vi "PH_Beckhoff_PPMA-Rods.panel.vi"(0 "object ref":refnum<vi>, 5 "error in (no error)":errorcluster) -> (19 "error out":errorcluster)   [LabVIEW 2014, in "PH_Beckhoff_PPMA-Rods.lvlib"]
doc: "This a GUI.\n\nLicense Agreement for this software:\n\nCopyright (C)\nGesellschaft für Schwerionenforschung, GSI\nPlanckstr. 1\n64291 Darmstadt\nGermany\n\nContact: D.Beck@gsi.de \n\nThis program is free software; you can redistribute it and/or modify it under the terms of the GNU General Public License as published by the Free Software Foundation; either version 2 of the license, or (at your option) any later version.\n\nThis program is distributed in the hope that it will be useful, but WITHOUT ANYW ARRANTY; without even the implied warranty of MERCHANTABILITY or FITNESS FOR A PARTICULAR PURPOSE. See the GNU General License for more details (http://www.gnu.org).\n\nGesellschaft für Schwerionenforschung, GSI\nPlanckstr. 1, 64291 Darmstadt, Germany\nFor all questions and ideas contact: M.Richter@gsi.de, H.Brand@gsi.de or D.Beck@gsi.de.\nLast update: 18-DEC-2002"
uses:
  PH_Beckhoff_PPMA-Rods.lvlib
  PH_Beckhoff/PH_Beckhoff.Connectivity.ctl
  PH_Beckhoff/PH_Beckhoff.ADS Error.ctl
  PH_Beckhoff/PH_Beckhoff.Values.ctl
  PH_Beckhoff/PH_Beckhoff.Sonderklemmen Inputs.ctl
  PH_Beckhoff/PH_Beckhoff.Analog Inputs.ctl
  PH_Beckhoff/PH_Beckhoff.Scaling Type.ctl
  PH_Beckhoff/PH_Beckhoff.Analog Outputs.ctl
  PH_Beckhoff/PH_Beckhoff.Digital Inputs.ctl
  PH_Beckhoff/PH_Beckhoff.Digital Outputs.ctl
  PH_Basics/PH_StatusHandler/PH_StatusHandler.GUI element.ctl
  PH_Beckhoff/PH_Beckhoff.GUI Refs.ctl
  CS_Core/CSObj/CSObj.lvlib
  PH_Basics/PH_Common/PH_Common.lvlib
  PH_Beckhoff/PH_Beckhoff.lvlib
  CS_Core/CSSystem/CSSystemLib/CSSystemLib.lvlib
  PH_Basics/PH_Class/PH_Class.lvlib
  PH_Basics/PH_StatusHandler/PH_StatusHandler.lvlib
panel:
  in  "Tab Control":enum32{"Beckhoff Stuff", "Rods ..."}(tab)=enum."Rods ..."
  out "Current Values":T1
  out "ADS Error":T8
  out "IP":string
  out "Connection":T9
  out "configured?":bool
  out "Prdc Int [ms]":i32
  out "valve closed":u32(colorbox)
  out "door locked K2":u32(colorbox)
  out "door locked K1":u32(colorbox)
  out "earth ok":u32(colorbox)
  in  "Warnlamp green on":bool
  in  "Warnlamp orange on":bool
  out "PILC":T10 caption="Enabling State"
  out "FR":T10 caption="Enabling State"
  out "PU 6":T10 caption="Enabling State"
  out "PU 5":T10 caption="Enabling State"
  out "PU 4":T10 caption="Enabling State"
  out "PU 3":T10 caption="Enabling State"
  out "PU 2":T10 caption="Enabling State"
  out "PU 1":T10 caption="Enabling State"
  out "ROD 51":u32(colorbox)
  out "ROD 53":u32(colorbox)
  out "ROD 52":u32(colorbox)
  out "ROD 54":u32(colorbox)
  out "ROD 50":u32(colorbox)
  out "ROD 49":u32(colorbox)
  out "ROD 48":u32(colorbox)
  out "ROD 47":u32(colorbox)
  out "ROD 46":u32(colorbox)
  out "ROD 45":u32(colorbox)
  out "ROD 44":u32(colorbox)
  out "ROD 43":u32(colorbox)
  out "ROD 42":u32(colorbox)
  out "ROD 41":u32(colorbox)
  out "ROD 39":u32(colorbox)
  out "ROD 40":u32(colorbox)
  out "ROD 37":u32(colorbox)
  out "ROD 38":u32(colorbox)
  out "ROD 35":u32(colorbox)
  out "ROD 36":u32(colorbox)
  out "ROD 33":u32(colorbox)
  out "ROD 34":u32(colorbox)
  out "ROD 31":u32(colorbox)
  out "ROD 32":u32(colorbox)
  out "ROD 30":u32(colorbox)
  out "ROD 29":u32(colorbox)
  out "ROD 28":u32(colorbox)
  out "ROD 27":u32(colorbox)
  out "ROD 26":u32(colorbox)
  out "ROD 25":u32(colorbox)
  out "ROD 24":u32(colorbox)
  out "ROD 23":u32(colorbox)
  out "ROD 22":u32(colorbox)
  out "ROD 21":u32(colorbox)
  out "ROD 19":u32(colorbox)
  out "ROD 20":u32(colorbox)
  out "ROD 17":u32(colorbox)
  out "ROD 18":u32(colorbox)
  out "ROD 15":u32(colorbox)
  out "ROD 16":u32(colorbox)
  out "ROD 13":u32(colorbox)
  out "ROD 14":u32(colorbox)
  out "ROD 11":u32(colorbox)
  out "ROD 12":u32(colorbox)
  out "ROD 10":u32(colorbox)
  out "ROD 9":u32(colorbox)
  out "ROD 8":u32(colorbox)
  out "ROD 7":u32(colorbox)
  out "ROD 6":u32(colorbox)
  out "ROD 5":u32(colorbox)
  out "ROD 4":u32(colorbox)
  out "ROD 3":u32(colorbox)
  out "ROD 2":u32(colorbox)
  out "ROD 1":u32(colorbox)
  in  "rods_chain_b_up":bool
  in  "rods_chain_a_up":bool
  in  "Show Info":bool
  in  "Delete":bool
  in  "Exit":bool
  # "PCS"
  # "3.40"
  # "Pay attention! Commands are remote controlled! Handle with care!"
  # "B"
  # "A"
  # "B"
  # "A"
  # "A"
  # "B"
  # "B"
  # "A"
  # "A"
  # "B"
  # "A"
  # "B"
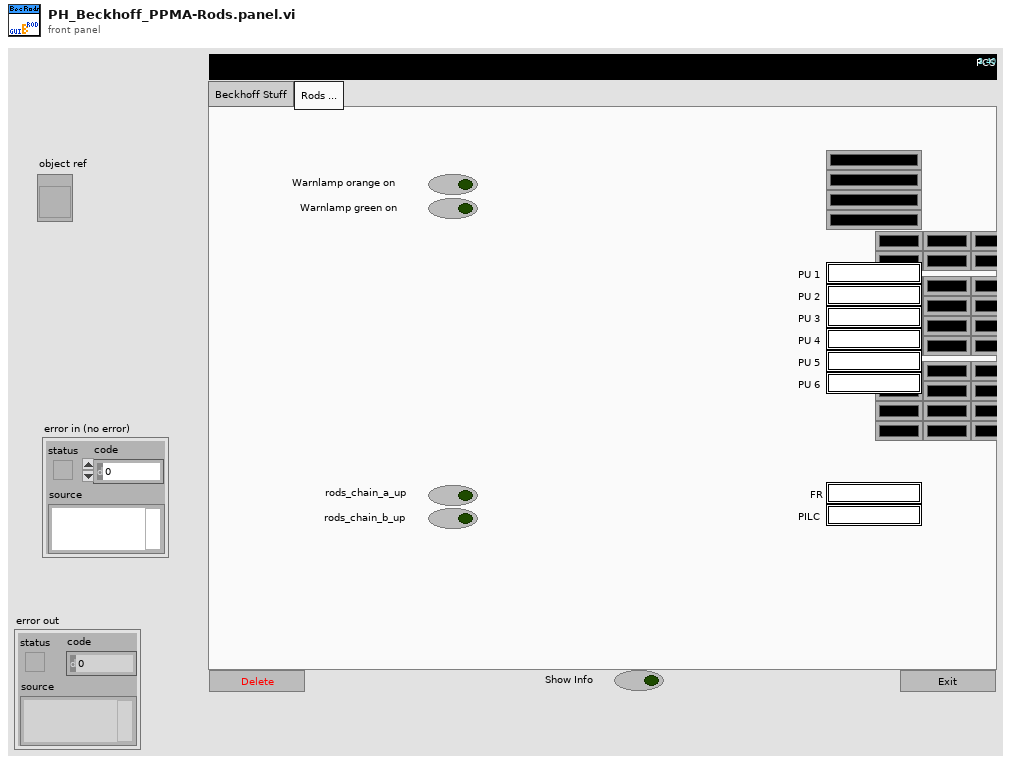
[diagram p1: front panel]
types:
  T1 = typedef "PH_Beckhoff.lvlib/PH_Beckhoff.Values.ctl" = cluster{"Sonderklemmen Inputs":T2, "Analog Inputs":T3, "Analog Outputs":T5, "Digital Inputs":T6, "Digital Outputs":T7}
  T2 = typedef "PH_Beckhoff.lvlib/PH_Beckhoff.Sonderklemmen Inputs.ctl" = cluster{"Total Length":u32, "Name":string, "Value":u64, "Quality":bool, "Service ID":i32, "Offset":u32, "Length":u32}[]
  T3 = typedef "PH_Beckhoff.lvlib/PH_Beckhoff.Analog Inputs.ctl" = cluster{"Name":string, "Value":u32, "Quality":bool, "Service ID":i32, "Sca Type":T4}[]
  T4 = typedef "PH_Beckhoff.lvlib/PH_Beckhoff.Scaling Type.ctl" = enum16{"none", "0 ... 15 Bit -> 0 ... 5", "0 ... 15 Bit -> 0 ... 10", "0 ... 15 Bit -> 0 ... 25", "0 ... 15 Bit -> 4 ... 20", "0 ... 15 Bit -> 0 ... 1", "0 ... 15 Bit -> 0 ... 20000", "0 ... 15 Bit -> 0 ... 24000"}
  T5 = typedef "PH_Beckhoff.lvlib/PH_Beckhoff.Analog Outputs.ctl" = cluster{"Name":string, "Value":u32, "Quality":bool, "Wanted Value":u32, "Service ID":i32, "Sca Type":T4}[]
  T6 = typedef "PH_Beckhoff.lvlib/PH_Beckhoff.Digital Inputs.ctl" = cluster{"Name":string, "Value":bool, "Quality":bool, "Service ID":i32, "inverted?":bool}[]
  T7 = typedef "PH_Beckhoff.lvlib/PH_Beckhoff.Digital Outputs.ctl" = cluster{"Name":string, "Value":bool, "Quality":bool, "Wanted Value":bool, "Service ID":i32, "inverted?":bool}[]
  T8 = typedef "PH_Beckhoff.lvlib/PH_Beckhoff.ADS Error.ctl" = cluster{"Latest Error":string, "Error List":string[]}
  T9 = typedef "PH_Beckhoff.lvlib/PH_Beckhoff.Connectivity.ctl" = cluster{"DLL?":bool, "Port?":bool, "Client?":bool, "Ping?":bool, "unsuccessful Pings":u32}
  T10 = typedef "PH_StatusHandler.lvlib/PH_StatusHandler.GUI element.ctl" = u16
  T11 = typedef "PH_Beckhoff.lvlib/PH_Beckhoff.GUI Refs.ctl" = cluster{"ADS Error":refnum<vi>, "Values":refnum<vi>, "configured?":refnum<vi>, "Connection":refnum<vi>, "IP":refnum<vi>, "Prdc Int [ms]":refnum<vi>}
  T12 = typedef "PH_Beckhoff.lvlib/PH_Beckhoff.i attribute.ctl" = cluster{"GUI Refs":T11, "operation?":bool, "Default Prdc Interval":i32, "Connection":T9, "AMS Net ID":T13, "Klemmencluster: # of":T14, "Values":T1, "IP":string, "Description":string, "configured?":bool, "Change Manager":cluster{"Detemination wanted?":bool, "Values changed at":cluster{"Sonderklemmen Inputs":i32[], "Analog Inputs":i32[], "Analog Outputs":i32[], "Digital Inputs":i32[], "Digital Outputs":i32[]}}, "Difference to handle an analog input as change":u32}
  T13 = typedef "Beckhoff - Driver np.lvlib/Beckhoff Access.ctl" = cluster{"DLL path":path, "AMS Net ID":cluster{"1st # of IP":u8, "2nd # of IP":u8, "3rd # of IP":u8, "4th # of IP":u8, "In Port":u8, "Out Port":u8}}
  T14 = typedef "Beckhoff - Driver np.lvlib/Klemmendeclarer.ctl" = cluster{"Offset due to Sonderklemms":u32, "analog Inputs":u32, "analog Outputs":u32, "digital Input Bits":u32, "digital Output Bits":u32}
  T15 = typedef "PH_Beckhoff_PPMA-Rods.lvlib/PH_Beckhoff_PPMA-Rods.i attribute.ctl" = cluster{"Input Up GUI Refs":refnum<vi>[], "Output GUI Refs":cluster{"Rod A up":refnum<vi>, "Rod B up":refnum<vi>, "Warnlamp orange":refnum<vi>, "Warnlamp green":refnum<vi>}, "States":cluster{"GUI Ref":refnum<vi>, "Status":T16, "Service ID":i32}[], "Input GUI Refs":cluster{"earth ok":refnum<vi>, "door locked K1":refnum<vi>, "door locked K2":refnum<vi>, "valve closed":refnum<vi>}}
  T16 = typedef "PH_StatusHandler.lvlib/PH_StatusHandler.Status.ctl" = i16
  T17 = cluster{"GUI Ref":refnum<vi>, "Status":T16, "Service ID":i32}[]
  T18 = cluster{"GUI Ref":refnum<vi>, "Status":T16, "Service ID":i32}
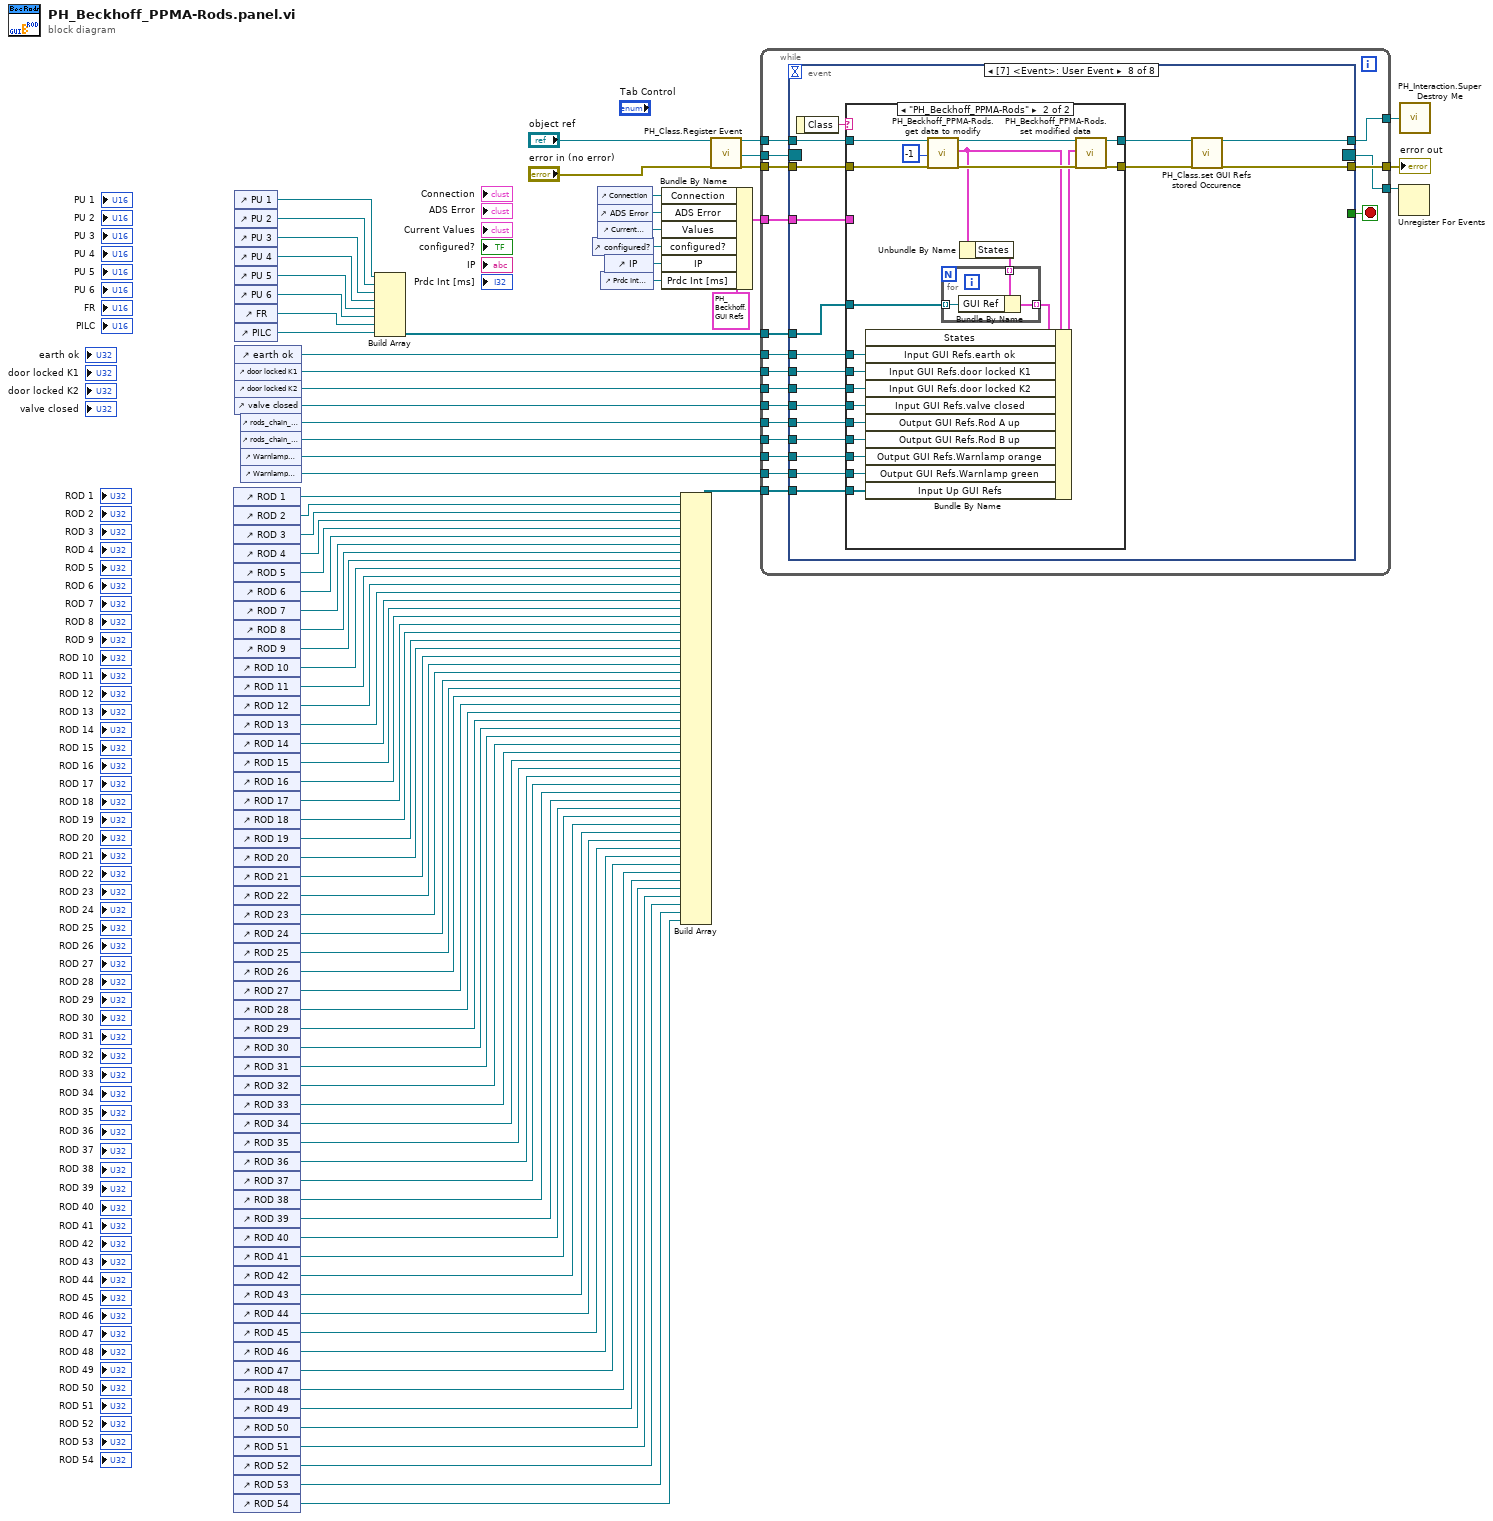
[diagram p0: block diagram]
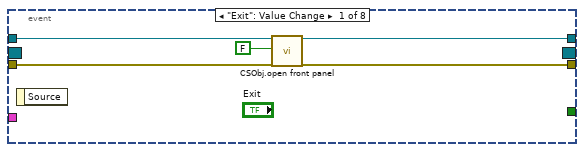
[diagram p2: hidden frame]
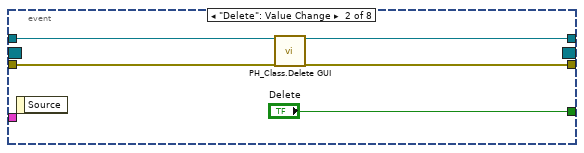
[diagram p3: hidden frame]
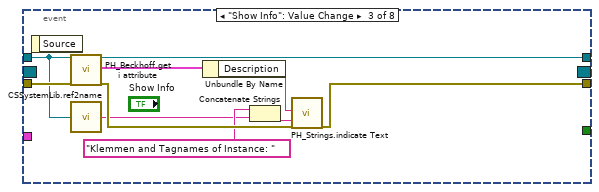
[diagram p4: hidden frame]
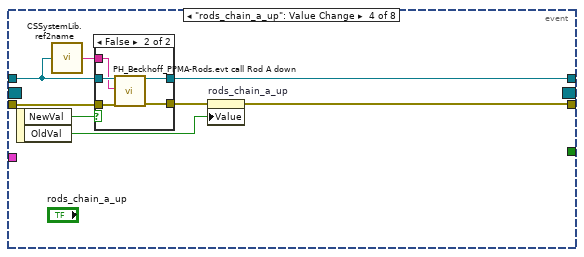
[diagram p5: hidden frame]
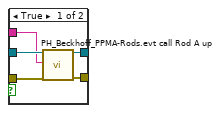
[diagram p6: hidden frame]
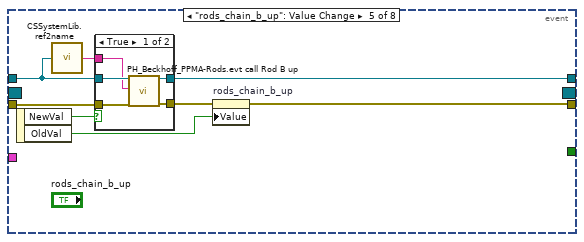
[diagram p7: hidden frame]
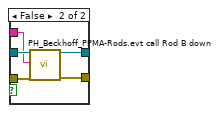
[diagram p8: hidden frame]
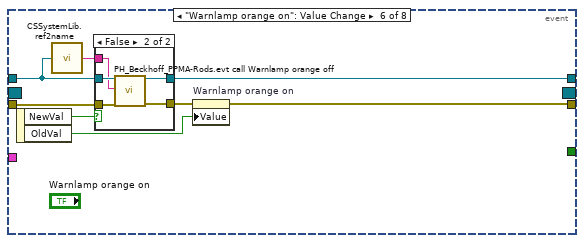
[diagram p9: hidden frame]
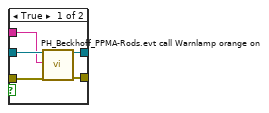
[diagram p10: hidden frame]
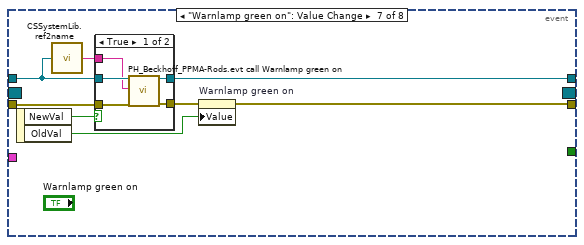
[diagram p11: hidden frame]
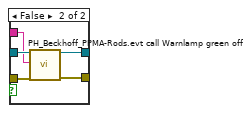
[diagram p12: hidden frame]
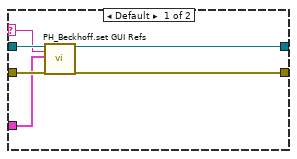
[diagram p13: hidden frame]
diagram:
  n1 = control-ref of="ROD 1"() -> (w81:refnum<vi>)
  n2 = control-ref of="ROD 2"() -> (w80:refnum<vi>)
  n3 = control-ref of="ROD 3"() -> (w79:refnum<vi>)
  n4 = control-ref of="ROD 4"() -> (w78:refnum<vi>)
  n5 = control-ref of="ROD 5"() -> (w77:refnum<vi>)
  n6 = control-ref of="ROD 6"() -> (w76:refnum<vi>)
  n7 = control-ref of="ROD 7"() -> (w75:refnum<vi>)
  n8 = control-ref of="ROD 8"() -> (w74:refnum<vi>)
  n9 = control-ref of="ROD 9"() -> (w73:refnum<vi>)
  n10 = control-ref of="ROD 10"() -> (w72:refnum<vi>)
  n11 = control-ref of="ROD 11"() -> (w71:refnum<vi>)
  n12 = control-ref of="ROD 12"() -> (w70:refnum<vi>)
  n13 = control-ref of="ROD 13"() -> (w69:refnum<vi>)
  n14 = control-ref of="ROD 14"() -> (w68:refnum<vi>)
  n15 = control-ref of="ROD 15"() -> (w67:refnum<vi>)
  n16 = control-ref of="ROD 16"() -> (w66:refnum<vi>)
  n17 = control-ref of="ROD 17"() -> (w65:refnum<vi>)
  n18 = control-ref of="ROD 18"() -> (w64:refnum<vi>)
  n19 = control-ref of="ROD 19"() -> (w63:refnum<vi>)
  n20 = control-ref of="ROD 20"() -> (w62:refnum<vi>)
  n21 = control-ref of="ROD 21"() -> (w61:refnum<vi>)
  n22 = control-ref of="ROD 22"() -> (w60:refnum<vi>)
  n23 = control-ref of="ROD 23"() -> (w59:refnum<vi>)
  n24 = control-ref of="ROD 24"() -> (w58:refnum<vi>)
  n25 = control-ref of="ROD 25"() -> (w57:refnum<vi>)
  n26 = control-ref of="ROD 26"() -> (w56:refnum<vi>)
  n27 = control-ref of="ROD 27"() -> (w55:refnum<vi>)
  n28 = control-ref of="ROD 28"() -> (w54:refnum<vi>)
  n29 = control-ref of="ROD 29"() -> (w53:refnum<vi>)
  n30 = control-ref of="ROD 30"() -> (w52:refnum<vi>)
  n31 = control-ref of="ROD 31"() -> (w51:refnum<vi>)
  n32 = control-ref of="ROD 32"() -> (w50:refnum<vi>)
  n33 = control-ref of="ROD 33"() -> (w49:refnum<vi>)
  n34 = control-ref of="ROD 34"() -> (w48:refnum<vi>)
  n35 = control-ref of="ROD 35"() -> (w47:refnum<vi>)
  n36 = control-ref of="ROD 36"() -> (w46:refnum<vi>)
  n37 = control-ref of="ROD 37"() -> (w45:refnum<vi>)
  n38 = control-ref of="ROD 38"() -> (w44:refnum<vi>)
  n39 = control-ref of="ROD 39"() -> (w43:refnum<vi>)
  n40 = control-ref of="ROD 40"() -> (w42:refnum<vi>)
  n41 = control-ref of="ROD 41"() -> (w41:refnum<vi>)
  n42 = control-ref of="ROD 42"() -> (w40:refnum<vi>)
  n43 = control-ref of="ROD 43"() -> (w39:refnum<vi>)
  n44 = control-ref of="ROD 44"() -> (w38:refnum<vi>)
  n45 = control-ref of="ROD 45"() -> (w37:refnum<vi>)
  n46 = control-ref of="ROD 46"() -> (w36:refnum<vi>)
  n47 = control-ref of="ROD 47"() -> (w35:refnum<vi>)
  n48 = control-ref of="ROD 48"() -> (w34:refnum<vi>)
  n49 = control-ref of="ROD 49"() -> (w33:refnum<vi>)
  n50 = control-ref of="ROD 50"() -> (w32:refnum<vi>)
  n51 = control-ref of="ROD 51"() -> (w31:refnum<vi>)
  n52 = control-ref of="ROD 52"() -> (w30:refnum<vi>)
  n53 = control-ref of="ROD 53"() -> (w29:refnum<vi>)
  n54 = control-ref of="ROD 54"() -> (w28:refnum<vi>)
  n55 = control-ref of="PU 1"() -> (w1:refnum<vi>)
  n56 = control-ref of="PU 2"() -> (w2:refnum<vi>)
  n57 = control-ref of="PU 3"() -> (w3:refnum<vi>)
  n58 = control-ref of="PU 4"() -> (w4:refnum<vi>)
  n59 = control-ref of="PU 5"() -> (w5:refnum<vi>)
  n60 = control-ref of="PU 6"() -> (w6:refnum<vi>)
  n61 = control-ref of="FR"() -> (w7:refnum<vi>)
  n62 = control-ref of="PILC"() -> (w8:refnum<vi>)
  n63 = control-ref of="earth ok"() -> (w22:refnum<vi>)
  n64 = control-ref of="door locked K1"() -> (w21:refnum<vi>)
  n65 = control-ref of="door locked K2"() -> (w20:refnum<vi>)
  n66 = control-ref of="valve closed"() -> (w19:refnum<vi>)
  n67 = control-ref of="rods_chain_a_up"() -> (w18:refnum<vi>)
  n68 = control-ref of="rods_chain_b_up"() -> (w17:refnum<vi>)
  n69 = control-ref of="Warnlamp orange on"() -> (w16:refnum<vi>)
  n70 = control-ref of="Warnlamp green on"() -> (w15:refnum<vi>)
  n71 = Build Array(w1, w2, w3, w4, w5, w6, w7, w8) -> (w23:refnum<vi>[])
  n72 = control-ref of="configured?"() -> (w82:refnum<vi>)
  n73 = control-ref of="Connection"() -> (w86:refnum<vi>)
  n74 = control-ref of="ADS Error"() -> (w85:refnum<vi>)
  n75 = control-ref of="Current Values"() -> (w83:refnum<vi>)
  n76 = control-ref of="Prdc Int [ms]"() -> (w9:refnum<vi>)
  n77 = control-ref of="IP"() -> (w10:refnum<vi>)
  n78 = Bundle By Name(cluster=T11 {"ADS Error"=refnum, "Values"=refnum, "configured?"=refnum, "Connection"=refnum, "IP"=refnum, "Prdc Int [ms]"=refnum} ("GUI Refs"), "Connection"=w86, "ADS Error"=w85, "Values"=w83, "configured?"=w82, "IP"=w10, "Prdc Int [ms]"=w9) -> (w13:T11)
  n79 = Build Array(w81, w80, w79, w78, w77, w76, w75, w74, w73, w72, w71, w70, w69, w68, w67, w66, w65, w64, w63, w62, w61, w60, w59, w58, w57, w56, w55, w54, w53, w52, w51, w50, w49, w48, w47, w46, w45, w44, w43, w42, w41, w40, w39, w38, w37, w36, w35, w34, w33, w32, w31, w30, w29, w28) -> (w14:refnum<vi>[])
  n80 = call "PH_Class.Register Event.vi"("i ref in"="object ref", "error in (no error)"="error in (no error)") -> ("i ref out"=w27:refnum<vi>, "Event Registration Refnum"=w25:refnum<event-registration>, "error out"=w26:errorcluster)  [unwired: 15 in]
  n81 = while {
    tunnel: w27 -> [w103]
    tunnel: [w102] -> w88
    tunnel: w26 -> [w105]
    tunnel: [w104] -> w87
    tunnel: w25 -> [w101]
    tunnel: [w100] -> w24
    tunnel: w23 -> [w99]
    tunnel: w22 -> [w98]
    tunnel: w21 -> [w97]
    tunnel: w20 -> [w96]
    tunnel: w19 -> [w95]
    tunnel: w18 -> [w94]
    tunnel: w17 -> [w93]
    tunnel: w16 -> [w92]
    tunnel: w15 -> [w91]
    tunnel: w14 -> [w90]
    tunnel: w13 -> [w89]
    stop <- w106 stop-if-true
    n82 = event shown="[7] <Event>: User Event" {
      selector: w101 -> [_ _ _ _ _ _ _ _]
      dyn-events: [_ _ _ _ _ _ _ _] -> w100
      timeout: _ -> [_ _ _ _ _ _ _ _]
      tunnel: [_ "Delete" _ _ _ _ _ _] -> w106
      tunnel: w103 -> [w108 w113 w117 w132 w150 w168 w186 w216]
      tunnel: w105 -> [w111 w115 w126 w134 w152 w170 w188 w205]
      tunnel: [w110 w114 w123 w129 w146 w163 w182 w201] -> w104
      tunnel: [w107 w112 w125 w133 w151 w169 w187 w199] -> w102
      tunnel: w99 -> [_ _ _ _ _ _ _ w215]
      tunnel: w98 -> [_ _ _ _ _ _ _ w214]
      tunnel: w97 -> [_ _ _ _ _ _ _ w213]
      tunnel: w96 -> [_ _ _ _ _ _ _ w212]
      tunnel: w95 -> [_ _ _ _ _ _ _ w211]
      tunnel: w94 -> [_ _ _ _ _ _ _ w210]
      tunnel: w93 -> [_ _ _ _ _ _ _ w209]
      tunnel: w92 -> [_ _ _ _ _ _ _ w208]
      tunnel: w91 -> [_ _ _ _ _ _ _ w207]
      tunnel: w90 -> [_ _ _ _ _ _ _ w206]
      tunnel: w89 -> [_ _ _ _ _ _ _ w202]
      event "Exit": Value Change {
        n83 = event-data() -> ()  [unwired: 1 in, 1 out]
        n84 = call "CSObj.open front panel.vi"("i ref in"=w108, "frontPanelOpen"=FALSE ("front panel open"), "error in (no error)"=w111) -> ("i ref out"=w107:refnum<vi>, "error out"=w110:errorcluster)  [unwired: 15 in]
      }
      event "Delete": Value Change {
        n85 = event-data() -> ()  [unwired: 1 in, 1 out]
        n86 = call "PH_Class.Delete GUI.vi"("VI in"=w113, "error in (no error)"=w115) -> ("VI out"=w112:refnum<vi>, "error out"=w114:errorcluster)  [unwired: 16 in]
      }
      event "Show Info": Value Change {
        n87 = event-data() -> ()  [unwired: 1 in, 1 out]
        n88 = call "PH_Beckhoff.get i attribute.vi"("i ref in"=w117, "error in (no error)"=w126) -> ("i ref out"=w125:refnum<vi>, "i attribute"=w122:T12, "error out"=w124:errorcluster)  [unwired: 15 in]
        n89 = call "CSSystemLib.ref2name.vi"("obj refnum"=w117) -> ("name"=w118:string)
        n90 = Unbundle By Name(w122) -> ("Description"=w121:string)
        n91 = Concatenate Strings("Klemmen and Tagnames of Instance: " ("Caption.Text"), w118) -> (w119:string)
        n92 = call "PH_Strings.indicate Text.vi"("String to show"=w121, "Caption.Text"=w119, "error in (no error)"=w124) -> ("error out"=w123:errorcluster)  [unwired: 16 in]
      }
      event "rods_chain_a_up": Value Change {
        n93 = event-data() -> ("NewVal"=w130:bool, "OldVal"=w127:bool)  [unwired: 1 in]
        n94 = call "CSSystemLib.ref2name.vi"("obj refnum"=w132) -> ("name"=w131:string)
        n95 = case shown="False" w130 {
          tunnel: w134 -> [w139 w144]
          tunnel: [w138 w143] -> w133
          tunnel: w132 -> [w137 w142]
          tunnel: [w136 w141] -> w128
          tunnel: w131 -> [w135 w140]
          frame True {
            n96 = call "PH_Beckhoff_PPMA-Rods.evt call Rod A up.vi"("i ref in"=w137, "Instance name"=w135, "error in"=w139) -> ("i ref out"=w138:refnum<vi>, "error out"=w136:errorcluster)  [unwired: 15 in]
          }
          frame False {
            n97 = call "PH_Beckhoff_PPMA-Rods.evt call Rod A down.vi"("i ref in"=w142, "Instance name"=w140, "error in"=w144) -> ("i ref out"=w143:refnum<vi>, "error out"=w141:errorcluster)  [unwired: 15 in]
          }
        }
        n98 = property on="rods_chain_a_up" class="Bool (strict)"(error in=w128, "Value"=w127) -> (error out=w129:errorcluster)  [unwired: 1 in, 1 out]
      }
      event "rods_chain_b_up": Value Change {
        n99 = event-data() -> ("NewVal"=w148:bool, "OldVal"=w145:bool)  [unwired: 1 in]
        n100 = call "CSSystemLib.ref2name.vi"("obj refnum"=w150) -> ("name"=w149:string)
        n101 = case shown="True" w148 {
          tunnel: w152 -> [w157 w162]
          tunnel: [w156 w161] -> w151
          tunnel: w150 -> [w155 w160]
          tunnel: [w154 w159] -> w147
          tunnel: w149 -> [w153 w158]
          frame True {
            n102 = call "PH_Beckhoff_PPMA-Rods.evt call Rod B up.vi"("i ref in"=w155, "Instance name"=w153, "error in"=w157) -> ("i ref out"=w156:refnum<vi>, "error out"=w154:errorcluster)  [unwired: 15 in]
          }
          frame False {
            n103 = call "PH_Beckhoff_PPMA-Rods.evt call Rod B down.vi"("i ref in"=w160, "Instance name"=w158, "error in"=w162) -> ("i ref out"=w161:refnum<vi>, "error out"=w159:errorcluster)  [unwired: 15 in]
          }
        }
        n104 = property on="rods_chain_b_up" class="Bool (strict)"(error in=w147, "Value"=w145) -> (error out=w146:errorcluster)  [unwired: 1 in, 1 out]
      }
      event "Warnlamp orange on": Value Change {
        n105 = event-data() -> ("NewVal"=w166:bool, "OldVal"=w165:bool)  [unwired: 1 in]
        n106 = call "CSSystemLib.ref2name.vi"("obj refnum"=w168) -> ("name"=w167:string)
        n107 = case shown="False" w166 {
          tunnel: w170 -> [w175 w180]
          tunnel: [w174 w179] -> w169
          tunnel: w168 -> [w173 w178]
          tunnel: [w172 w177] -> w164
          tunnel: w167 -> [w171 w176]
          frame True {
            n108 = call "PH_Beckhoff_PPMA-Rods.evt call Warnlamp orange on.vi"("i ref in"=w173, "Instance name"=w171, "error in"=w175) -> ("i ref out"=w174:refnum<vi>, "error out"=w172:errorcluster)  [unwired: 15 in]
          }
          frame False {
            n109 = call "PH_Beckhoff_PPMA-Rods.evt call Warnlamp orange off.vi"("i ref in"=w178, "Instance name"=w176, "error in"=w180) -> ("i ref out"=w179:refnum<vi>, "error out"=w177:errorcluster)  [unwired: 15 in]
          }
        }
        n110 = property on="Warnlamp orange on" class="Bool (strict)"(error in=w164, "Value"=w165) -> (error out=w163:errorcluster)  [unwired: 1 in, 1 out]
      }
      event "Warnlamp green on": Value Change {
        n111 = event-data() -> ("NewVal"=w184:bool, "OldVal"=w181:bool)  [unwired: 1 in]
        n112 = call "CSSystemLib.ref2name.vi"("obj refnum"=w186) -> ("name"=w185:string)
        n113 = case shown="True" w184 {
          tunnel: w188 -> [w193 w198]
          tunnel: [w192 w197] -> w187
          tunnel: w186 -> [w191 w196]
          tunnel: [w190 w195] -> w183
          tunnel: w185 -> [w189 w194]
          frame True {
            n114 = call "PH_Beckhoff_PPMA-Rods.evt call Warnlamp green on.vi"("i ref in"=w191, "Instance name"=w189, "error in"=w193) -> ("i ref out"=w192:refnum<vi>, "error out"=w190:errorcluster)  [unwired: 15 in]
          }
          frame False {
            n115 = call "PH_Beckhoff_PPMA-Rods.evt call Warnlamp green off.vi"("i ref in"=w196, "Instance name"=w194, "error in"=w198) -> ("i ref out"=w197:refnum<vi>, "error out"=w195:errorcluster)  [unwired: 15 in]
          }
        }
        n116 = property on="Warnlamp green on" class="Bool (strict)"(error in=w183, "Value"=w181) -> (error out=w182:errorcluster)  [unwired: 1 in, 1 out]
      }
      event User Event {
        n117 = event-data() -> ("Class"=w204:string)  [unwired: 1 in]
        n118 = case shown="\"PH_Beckhoff_PPMA-Rods\"" w204 {
          selector: w204 -> [w218 _]
          tunnel: w216 -> [w222 w236]
          tunnel: w215 -> [_ w235]
          tunnel: w214 -> [_ w234]
          tunnel: w213 -> [_ w233]
          tunnel: w212 -> [_ w232]
          tunnel: w211 -> [_ w231]
          tunnel: w210 -> [_ w230]
          tunnel: w209 -> [_ w229]
          tunnel: w208 -> [_ w228]
          tunnel: w207 -> [_ w227]
          tunnel: w206 -> [_ w226]
          tunnel: w205 -> [w221 w225]
          tunnel: [w220 w224] -> w200
          tunnel: [w219 w223] -> w203
          tunnel: w202 -> [w217 _]
          frame Default {
            n119 = call "PH_Beckhoff.set GUI Refs.vi"("i ref in"=w222, "Class"=w218, "GUI Refs"=w217, "error in"=w221) -> ("i ref out"=w220:refnum<vi>, "error out"=w219:errorcluster)  [unwired: 14 in]
          }
          frame "PH_Beckhoff_PPMA-Rods" {
            n120 = call "PH_Beckhoff_PPMA-Rods.get data to modify.vi"("i ref in"=w236, "ms timeout (10000)"=-1, "error in (no error)"=w225) -> ("i ref out"=w242:refnum<vi>, "i attribute"=w239:T15, "error out"=w243:errorcluster)  [unwired: 13 in, 1 out]
            n121 = Unbundle By Name(w239) -> ("States"=w238:T17)
            n122 = for {
              tunnel: w238 -> [w246] mode=indexing
              tunnel: w235 -> [w245] mode=indexing
              tunnel: [w244] -> w237 mode=indexing
              n123 = Bundle By Name(cluster=w246, "GUI Ref"=w245) -> (w244:T18)
            }
            n124 = Bundle By Name(cluster=w239, "States"=w237, "Input GUI Refs.earth ok"=w234, "Input GUI Refs.door locked K1"=w233, "Input GUI Refs.door locked K2"=w232, "Input GUI Refs.valve closed"=w231, "Output GUI Refs.Rod A up"=w230, "Output GUI Refs.Rod B up"=w229, "Output GUI Refs.Warnlamp orange"=w228, "Output GUI Refs.Warnlamp green"=w227, "Input Up GUI Refs"=w226) -> (w240:T15)
            n125 = call "PH_Beckhoff_PPMA-Rods.set modified data.vi"("i ref in"=w242, "i attribute"=w240, "error in (no error)"=w243) -> ("i ref out"=w224:refnum<vi>, "error out"=w223:errorcluster)  [unwired: 15 in]
          }
        }
        n126 = call "PH_Class.set GUI Refs stored Occurence.vi"("i ref in"=w200, "error in (no error)"=w203) -> ("i ref out"=w199:refnum<vi>, "error out"=w201:errorcluster)  [unwired: 16 in]
      }
    }
  }
  "error out" <- w87
  n127 = Unregister For Events(event registration refnum=w24) -> ()  [unwired: 1 in, 1 out]
  n128 = call "PH_Interaction.Super Destroy Me.vi"("i ref out"=w88) -> ()
